vi "Subvi counter up U16.vi"(8 "Clock":bool, 9 "Nmax":u16) -> (1 "Output":u16)   [LabVIEW 2017]
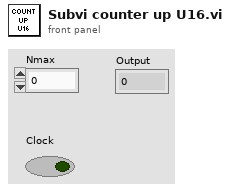
[diagram p1: front panel]
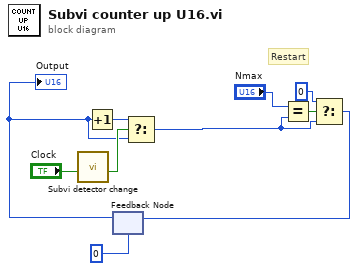
[diagram p0: block diagram]
diagram:
  # "Restart"
  n1 = call "Subvi detector change.vi"("Input"="Clock") -> ("Output"=w4:bool)  [unwired: 8 in]
  n2 = feedback #1(u16 0) -> (w1:u16)
  "Output" <- w1
  n3 = Increment(x=w1) -> (x+1=w3:u16)
  n4 = Select(t=w3, s=w4, f=w1) -> (s? t:f=w2:u16)
  n5 = Equal?(x="Nmax", y=w2) -> (x = y?=w10:bool)
  n6 = Select(t=u16 0, s=w10, f=w2) -> (s? t:f=w7:u16)
  n7 = feedback-in #1(w7) -> ()
